vi "Solve Complex Linear Equations (single right hand).vi"(2 "matrix type":T1, 3 "Known Vector":cdb[](array[numeric]) format="%.2f", 4 "Input Matrix":T2) -> (0 "error":i32, 1 "Solution Vector":cdb[](array[numeric]) format="%.2f")   [LabVIEW 2010, in "NI_AALPro.lvlib"]
doc: "Solves a linear system AX = Y. The data types you wire to the <B>Input Matrix</B> and <B>Known Vector</B> inputs determine the polymorphic instance to use."
uses:
  NI_AALPro.lvlib
  ComplexMatrix.ctl
  Matrix Type of Inverse Matrix.ctl
  Solve Complex Linear Eqs (Gen, single right hand).vi
  NI_AALBase.lvlib
  NI_Matrix.lvlib
panel:
  # "Solve Complex Linear Equations"
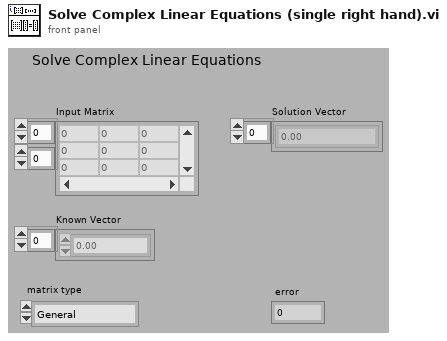
[diagram p1: front panel]
types:
  T1 = typedef "NI_AALBase.lvlib/Matrix Type of Inverse Matrix.ctl" = enum32{"General", "Positive Definite", "Lower Triangular", "Upper Triangular"}
  T2 = typedef "NI_Matrix.lvlib/ComplexMatrix.ctl" = cdb[][]
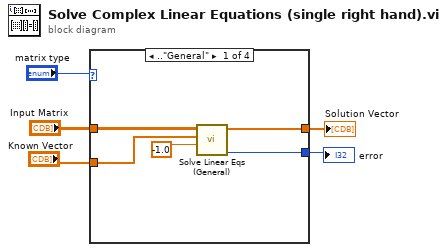
[diagram p0: block diagram]
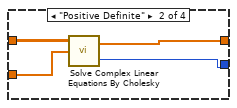
[diagram p2: hidden frame]
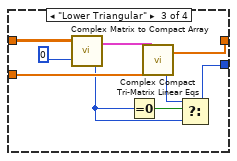
[diagram p3: hidden frame]
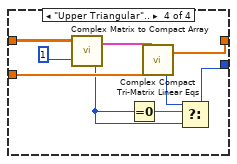
[diagram p4: hidden frame]
diagram:
  n1 = case shown="..\"General\"" "matrix type" {
    tunnel: "Known Vector" -> [w9 w11 w23 w32]
    tunnel: [w7 w12 w17 w24] -> w4
    tunnel: [w8 w13 w22 w31] -> w3
    tunnel: "Input Matrix" -> [w10 w14 w20 w29]
    frame .."General" {
      n2 = call-poly "Solve Linear Eqs (General).vi"("relative tolerance"=-1.0, "Known Vector"=w9, "Input Matrix"=w10) -> ("error"=w7:i32, "Solution Vector"=w8:cdb[])  [unwired: 7 in]
    }
    frame "Positive Definite" {
      n3 = call "Solve Complex Linear Equations By Cholesky.vi"("Known Vector"=w11, "Input Matrix"=w14) -> ("error"=w12:i32, "Solution Vector"=w13:cdb[])  [unwired: 1 in]
    }
    frame "Lower Triangular" {
      n4 = call "Complex Matrix to Compact Array.vi"("matrix type"=0, "Matrix A"=w20) -> ("error"=w16:i32, "Compact Array"=w19:cluster{"Compact Array":cdb[], "array type":i32})
      n5 = Equal To 0?(x=w16) -> (x = 0?=w18:bool)
      n6 = call "Complex Compact Tri-Matrix Linear Eqs.vi"("Known Vector"=w23, "Triangular Compact Array"=w19) -> ("error"=w15:i32, "Solution Vector"=w22:cdb[])
      n7 = Select(t=w15, s=w18, f=w16) -> (s? t:f=w17:i32)
    }
    frame "Upper Triangular".. {
      n8 = call "Complex Matrix to Compact Array.vi"("matrix type"=1, "Matrix A"=w29) -> ("error"=w26:i32, "Compact Array"=w28:cluster{"Compact Array":cdb[], "array type":i32})
      n9 = Equal To 0?(x=w26) -> (x = 0?=w27:bool)
      n10 = call "Complex Compact Tri-Matrix Linear Eqs.vi"("Known Vector"=w32, "Triangular Compact Array"=w28) -> ("error"=w25:i32, "Solution Vector"=w31:cdb[])
      n11 = Select(t=w25, s=w27, f=w26) -> (s? t:f=w24:i32)
    }
  }
  "error" <- w4
  "Solution Vector" <- w3
